vi "Write Channel.vi"(8 "error in (no error)":errorcluster, 10 "Channel":T1, 11 "Function Generator in":refnum<class "Function Generator.lvclass">) -> (0 "error out":errorcluster, 3 "Function Generator out":refnum<class "Function Generator.lvclass">)   [LabVIEW 2018, in "Function Generator.lvlib" / "Function Generator.lvclass"]
uses:
  Function Generator.lvclass
  Custom Controls/Channel.ctl
  Function Generator.lvclass/Function Generator.ctl
  Function Generator.lvlib
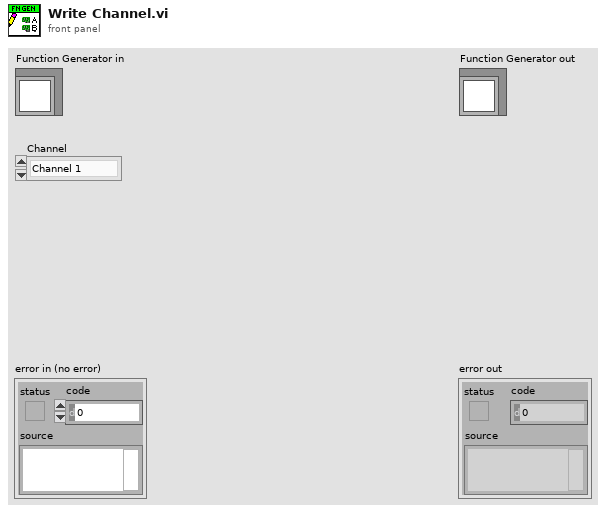
[diagram p1: front panel]
types:
  T1 = typedef "Function Generator.lvlib/Channel.ctl" = enum16{"Channel 1", "Channel 2", "Channel 3", "Channel 4"}
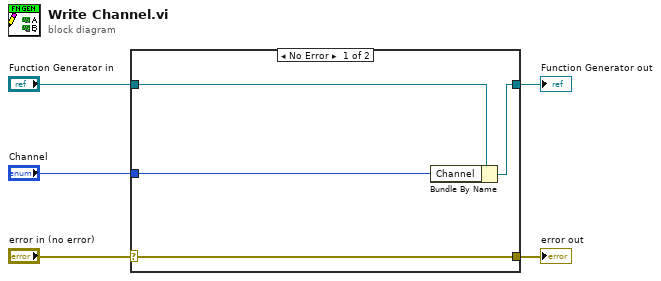
[diagram p0: block diagram]
diagram:
  n1 = case shown="No Error" "error in (no error)" {
    selector: "error in (no error)" -> [w9 w10]
    tunnel: [w9 w10] -> w4
    tunnel: [w7 w11] -> w2
    tunnel: "Function Generator in" -> [w8 w11]
    tunnel: "Channel" -> [w6 _]
    frame No Error {
      n2 = Bundle By Name(cluster=w8, "Channel"=w6) -> (w7:refnum<class "Function Generator.lvclass">)
    }
    frame Error {
    }
  }
  "error out" <- w4
  "Function Generator out" <- w2
